vi "sub vi - Manual Piezo.vi"() -> ()   [LabVIEW 2010]
uses:
  <vilib>/DAQmx/write.llb/DAQmx Write (Analog 1D DBL NChan 1Samp).vi
  <vilib>/DAQmx/create/channels.llb/DAQmx Create Channel (AO-Voltage-Basic).vi
  <vilib>/Utility/inputDevices.llb/keyboardAcquire.vi
  <vilib>/daqmx/miscellaneous.llb/DAQmx Fill In Error Info.vi
panel:
  out "appended array":dbl[](array[numeric])
  in  "stop 3":bool
  in  "Speed":dbl=1.0
  in  "wait time":u32=30
  out "Out of Piezo Range":bool
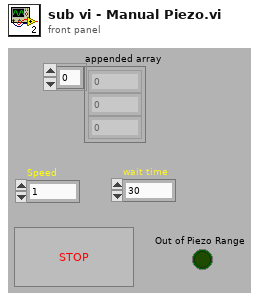
[diagram p1: front panel]
types:
  T1 = enum16{"0", "1", "2", "3", "4", "5", "6", "7", "8", "9", "A", "B", "C", "D", "E", "F", "G", "H", "I", "J", "K", "L", "M", "N", "O", "P", "Q", "R", "S", "T", "U", "V", "W", "X", "Y", "Z", "F1", "F2", "F3", "F4", "F5", "F6", "F7", "F8", "F9", "F10", "F11", "F12", "F13", "F14", "F15", "ADD", "BACK", "BACKSLASH", "CAPITAL", "COMMA", "DECIMAL", "DELETE", "DIVIDE", "DOWN", "END", "EQUALS", "ESCAPE", "GRAVE (`)", "HOME", "INSERT", "LBRACKET", "LCONTROL", "LEFT", "L ALT", "LSHIFT", "LWIN", "MINUS", "MULTIPLY", "NEXT", "NUMLOCK", "NUMPAD_0", "NUMPAD_1", "NUMPAD_2", "NUMPAD_3", "NUMPAD_4", "NUMPAD_5", "NUMPAD_6", "NUMPAD_7", "NUMPAD_8", "NUMPAD_9", "PAUSE", "PERIOD", "PRIOR (PG UP)", "RBRACKET", "RCONTROL", "RETURN", "RIGHT", "R ALT", "RSHIFT", "RWIN", "SCROLL", "SEMICOLON", "SLASH", "SPACE", "SUBTRACT", "TAB", "UP", "ENTER (num pad)", "' (quote)"}[]
  T2 = enum16{"0", "1", "2", "3", "4", "5", "6", "7", "8", "9", "A", "B", "C", "D", "E", "F", "G", "H", "I", "J", "K", "L", "M", "N", "O", "P", "Q", "R", "S", "T", "U", "V", "W", "X", "Y", "Z", "F1", "F2", "F3", "F4", "F5", "F6", "F7", "F8", "F9", "F10", "F11", "F12", "F13", "F14", "F15", "ADD", "BACK", "BACKSLASH", "CAPITAL", "COMMA", "DECIMAL", "DELETE", "DIVIDE", "DOWN", "END", "EQUALS", "ESCAPE", "GRAVE (`)", "HOME", "INSERT", "LBRACKET", "LCONTROL", "LEFT", "L ALT", "LSHIFT", "LWIN", "MINUS", "MULTIPLY", "NEXT", "NUMLOCK", "NUMPAD_0", "NUMPAD_1", "NUMPAD_2", "NUMPAD_3", "NUMPAD_4", "NUMPAD_5", "NUMPAD_6", "NUMPAD_7", "NUMPAD_8", "NUMPAD_9", "PAUSE", "PERIOD", "PRIOR (PG UP)", "RBRACKET", "RCONTROL", "RETURN", "RIGHT", "R ALT", "RSHIFT", "RWIN", "SCROLL", "SEMICOLON", "SLASH", "SPACE", "SUBTRACT", "TAB", "UP", "ENTER (num pad)", "' (quote)"}
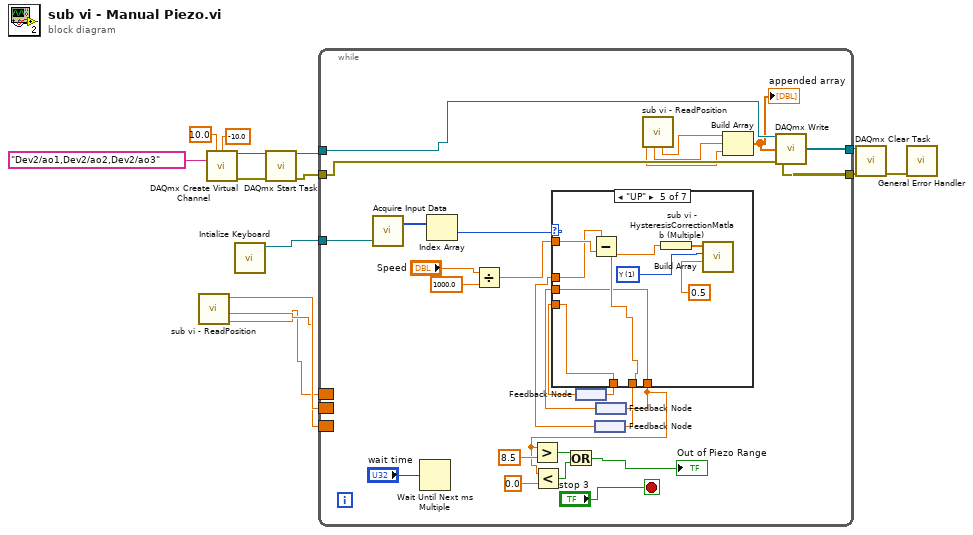
[diagram p0: block diagram]
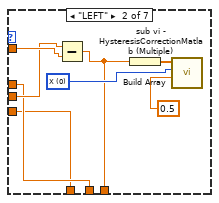
[diagram p3: hidden frame]
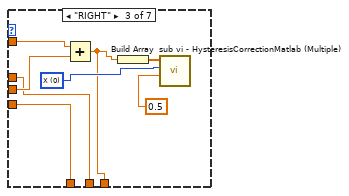
[diagram p4: hidden frame]
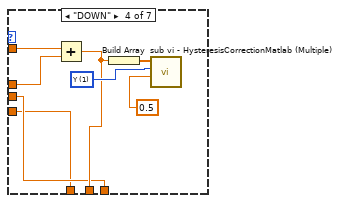
[diagram p5: hidden frame]
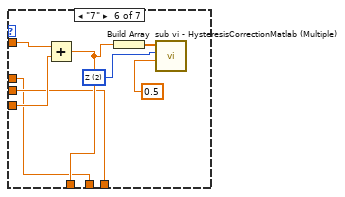
[diagram p6: hidden frame]
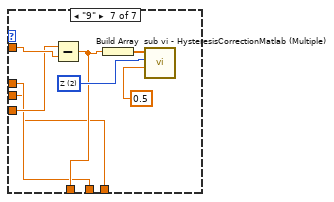
[diagram p7: hidden frame]
diagram:
  n1 = call "sub vi - ReadPosition.vi"() -> ("Z Position"=w1:dbl, "Y Position"=w2:dbl, "X Position"=w3:dbl)  [unwired: 9 out]
  n2 = call-poly <vilib>:"DAQmx Create Virtual Channel.vi"("maximum value"=10.0, "minimum value"=-10.0, "physical channels"=tag "Dev2/ao1,Dev2/ao2,Dev2/ao3") -> ("task out"=w6:refnum<k21>, "error out"=w5:errorcluster)  [unwired: 6 in, 5 out]
  n3 = call <vilib>:"Intialize Keyboard.vi"() -> ("device ID"=w12:refnum<k1>)  [unwired: 1 in, 10 out]
  n4 = call <vilib>:"DAQmx Start Task.vi"("task/channels in"=w6, "error in"=w5) -> ("task out"=w11:refnum<k21>, "error out"=w4:errorcluster)  [unwired: 12 out]
  n5 = while {
    tunnel: w12 -> [w38]
    tunnel: w11 -> [w19]
    tunnel: [w37] -> w10
    tunnel: [w36] -> w9
    tunnel: w4 -> [w20]
    border: w3 -> [_]
    border: w1 -> [_]
    border: w2 -> [_]
    stop <- "stop 3" stop-if-true
    n6 = call-poly <vilib>:"Acquire Input Data.vi"("device ID"=w38) -> ("keys pressed"=w41:T1)  [unwired: 1 in, 17 out]
    n7 = Wait Until Next ms Multiple(millisecond multiple="wait time") -> ()  [unwired: 1 out]
    n8 = Index Array(array=w41) -> (element=w39:T2)  [unwired: 1 in]
    n9 = Divide(x="Speed", y=1000.0) -> (x/y=w33:dbl)
    n10 = feedback #1() -> (w21:dbl)
    n11 = feedback #2() -> (w23:dbl)
    n12 = feedback #3() -> (w25:dbl)
    n13 = case shown="\"UP\"" w39 {
      tunnel: w33 -> [_ w52 w60 w68 w73 w84 w89]
      tunnel: [w42 w48 w56 w62 w69 w78 w85] -> w26
      tunnel: w25 -> [w42 w47 w55 w62 w69 w78 w85]
      tunnel: [w43 w46 w53 w64 w72 w77 w86] -> w24
      tunnel: w23 -> [w43 w46 w53 w63 w71 w77 w86]
      tunnel: [w44 w45 w54 w61 w70 w80 w88] -> w22
      tunnel: w21 -> [w44 w45 w54 w61 w70 w79 w87]
      frame "0", Default {
      }
      frame "LEFT" {
        w49 = u16 0 items=["X", "Y", "Z"] ("Axis")
        n14 = Subtract(x=w47, y=w52) -> (x-y=w48:dbl)
        n15 = Build Array(w48) -> (w50:dbl[])
        n16 = call "sub vi - HysteresisCorrectionMatlab (Multiple).vi"("frequency"=0.5, "Axis"=w49, "desired positions"=w50) -> ()  [unwired: 9 out]
      }
      frame "RIGHT" {
        w57 = u16 0 items=["X", "Y", "Z"] ("Axis")
        n17 = Add(x=w60, y=w55) -> (x+y=w56:dbl)
        n18 = Build Array(w56) -> (w58:dbl[])
        n19 = call "sub vi - HysteresisCorrectionMatlab (Multiple).vi"("frequency"=0.5, "Axis"=w57, "desired positions"=w58) -> ()  [unwired: 9 out]
      }
      frame "DOWN" {
        w65 = u16 1 items=["X", "Y", "Z"] ("Axis")
        n20 = Add(x=w68, y=w63) -> (x+y=w64:dbl)
        n21 = Build Array(w64) -> (w66:dbl[])
        n22 = call "sub vi - HysteresisCorrectionMatlab (Multiple).vi"("frequency"=0.5, "Axis"=w65, "desired positions"=w66) -> ()  [unwired: 9 out]
      }
      frame "UP" {
        w74 = u16 1 items=["X", "Y", "Z"] ("Axis")
        n23 = Subtract(x=w71, y=w73) -> (x-y=w72:dbl)
        n24 = Build Array(w72) -> (w75:dbl[])
        n25 = call "sub vi - HysteresisCorrectionMatlab (Multiple).vi"("frequency"=0.5, "Axis"=w74, "desired positions"=w75) -> ()  [unwired: 9 out]
      }
      frame "7" {
        w81 = u16 2 items=["X", "Y", "Z"] ("Axis")
        n26 = Add(x=w84, y=w79) -> (x+y=w80:dbl)
        n27 = Build Array(w80) -> (w82:dbl[])
        n28 = call "sub vi - HysteresisCorrectionMatlab (Multiple).vi"("frequency"=0.5, "Axis"=w81, "desired positions"=w82) -> ()  [unwired: 9 out]
      }
      frame "9" {
        w90 = u16 2 items=["X", "Y", "Z"] ("Axis")
        n29 = Subtract(x=w87, y=w89) -> (x-y=w88:dbl)
        n30 = Build Array(w88) -> (w91:dbl[])
        n31 = call "sub vi - HysteresisCorrectionMatlab (Multiple).vi"("frequency"=0.5, "Axis"=w90, "desired positions"=w91) -> ()  [unwired: 9 out]
      }
    }
    n32 = Greater?(x=w26, y=8.5) -> (0:w32:bool)
    n33 = Less?(x=w26, y=0.0) -> (x < y?=w31:bool)
    n34 = Or(x=w32, y=w31) -> (x .or. y?=→"Out of Piezo Range":bool)
    n35 = feedback-in #1(w22) -> ()
    n36 = feedback-in #2(w24) -> ()
    n37 = feedback-in #3(w26) -> ()
    n38 = call "sub vi - ReadPosition.vi"() -> ("X Voltage"=w18:dbl, "Y Voltage"=w17:dbl, "Z Voltage"=w16:dbl)  [unwired: 9 out]
    n39 = Build Array(w18, w17, w16) -> (w15:dbl[])
    "appended array" <- w15
    n40 = call-poly <vilib>:"DAQmx Write.vi"("task/channels in"=w19, "data"=w15, "error in"=w20) -> ("task out"=w37:refnum<k21>, "error out"=w36:errorcluster)  [unwired: 1 in, 10 out]
  }
  n41 = call <vilib>:"DAQmx Clear Task.vi"("task in"=w10, "error in"=w9) -> ("error out"=w7:errorcluster)  [unwired: 13 out]
  n42 = call <vilib>:"General Error Handler.vi"("error in (no error)"=w7) -> ()  [unwired: 1 in, 14 out]
